vi "Eurotherm_2023_Module.vi"(3 "SP":bool=TRUE, 4 "Decimales":u16(ring)=1 items=["0"=1, "1"=10, "2"=100], 5 "Eurotherm (T:Enable)":bool=TRUE, 7 "Command":T3, 8 "error in (no error)":errorcluster, 9 "Value":dbl format="%04.1g", 10 "Address":T1(ring), 11 "VISA resource name":refnum<visa-resource-name>) -> (0 "error out":errorcluster, 2 "Eurotherm":T2)   [LabVIEW 2017]
uses:
  Eurotherm_2023_Module.ctl
  <vilib>/Instr/_visa.llb/VISA Configure Serial Port (Instr).vi
panel:
  out "String Read":string
  out "String Write":string
  # "NUEVO MODULO VI\nQUE INCORPORA LÍMITES DE SALIDA"
  # "Eurotherm New Module"
  # "Input Data"
  # "Local Data"
  # "Output Data"
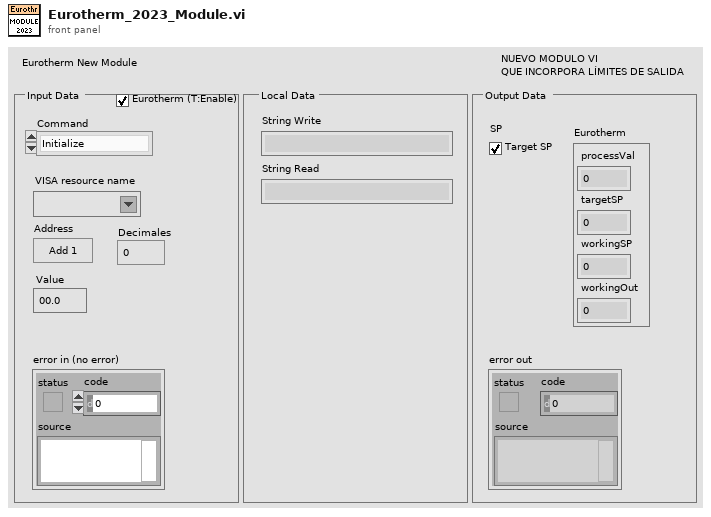
[diagram p1: front panel]
types:
  T1 = enum16{"Add 1", "Add 2", "Add 3", "Add 10", "Add 11", "Add 12", "Add 13"}
  T2 = cluster{"processVal":dbl, "targetSP":dbl, "workingSP":dbl, "workingOut":dbl}
  T3 = typedef "Eurotherm_2023_Module.ctl" = enum16{"Initialize", "Write setpoint", "Read data", "Write ramp rate", "Set constante proporcional", "Set constante integral", "Set constante diferencial", "Set ouput limit LOW", "Set ouput limit HIGH", "Shutdown"}
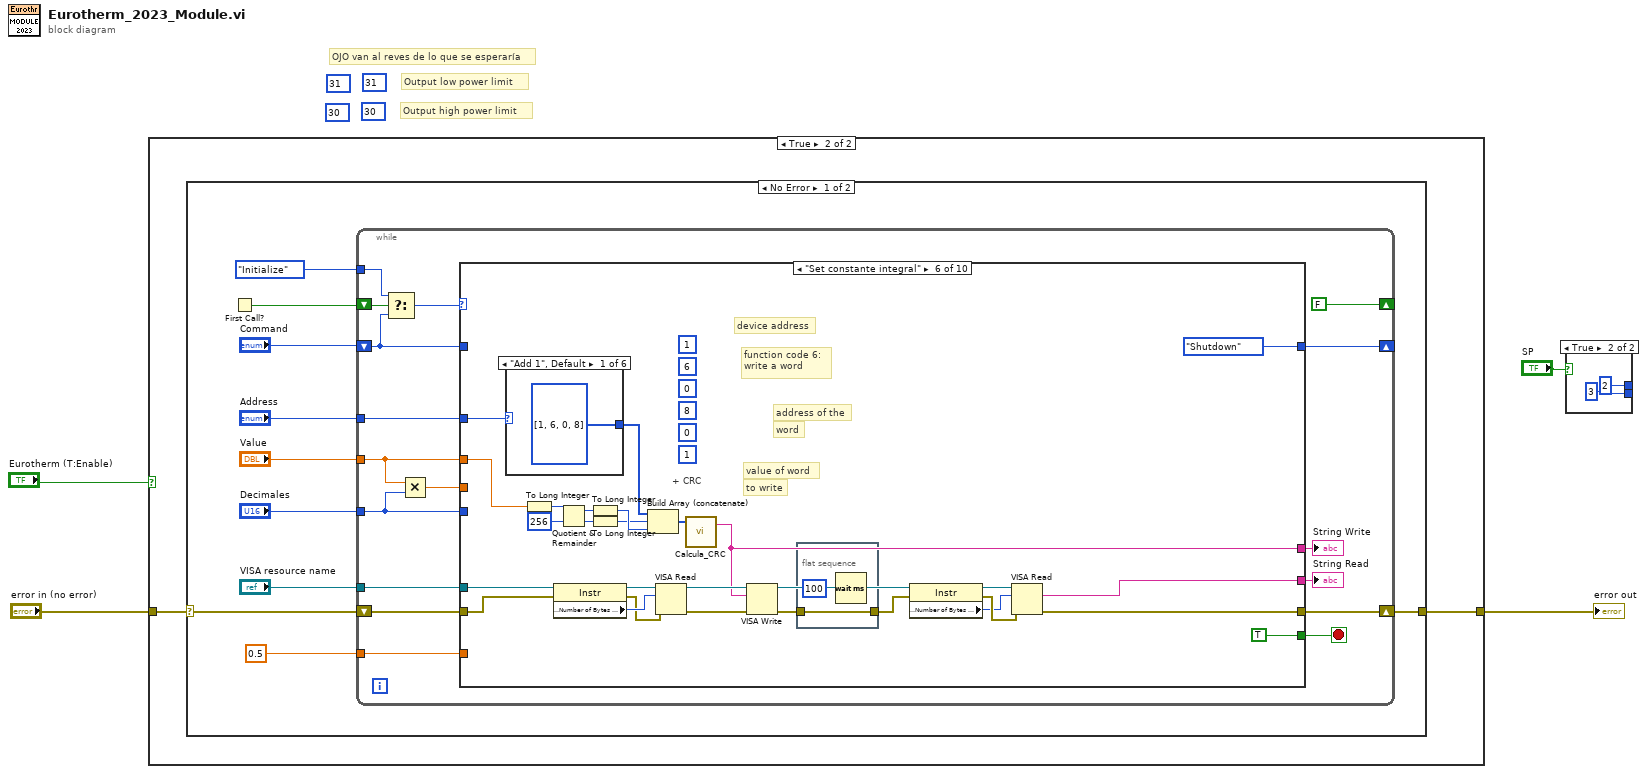
[diagram p0: block diagram]
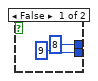
[diagram p2: hidden frame]
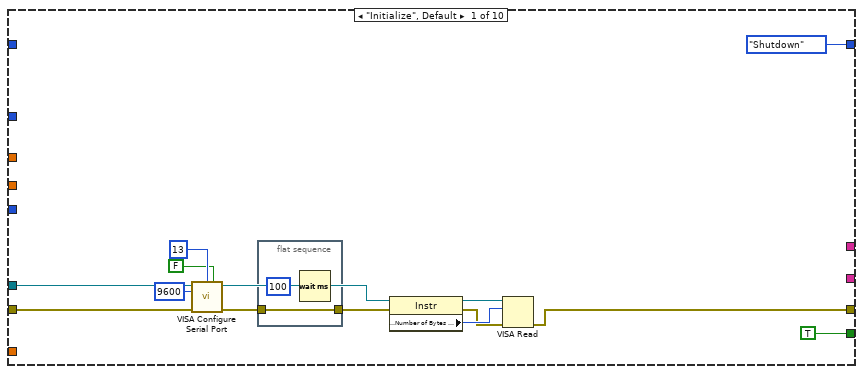
[diagram p4: hidden frame]
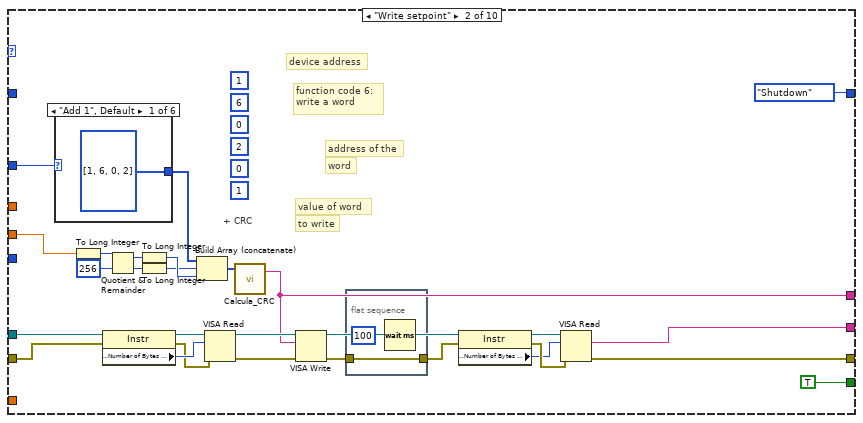
[diagram p5: hidden frame]
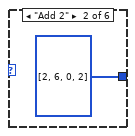
[diagram p6: hidden frame]
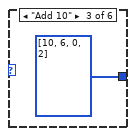
[diagram p7: hidden frame]
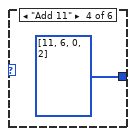
[diagram p8: hidden frame]
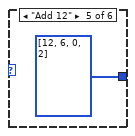
[diagram p9: hidden frame]
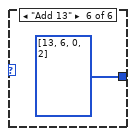
[diagram p10: hidden frame]
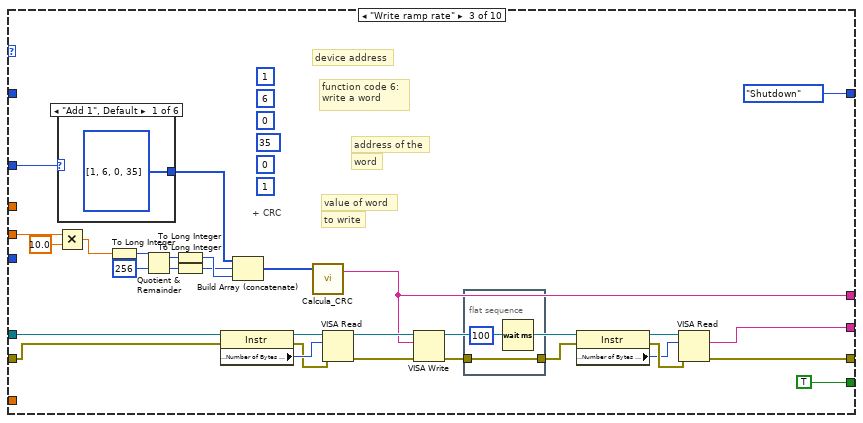
[diagram p11: hidden frame]
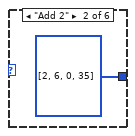
[diagram p12: hidden frame]
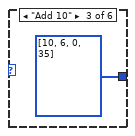
[diagram p13: hidden frame]
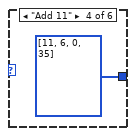
[diagram p14: hidden frame]
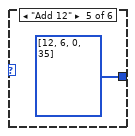
[diagram p15: hidden frame]
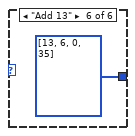
[diagram p16: hidden frame]
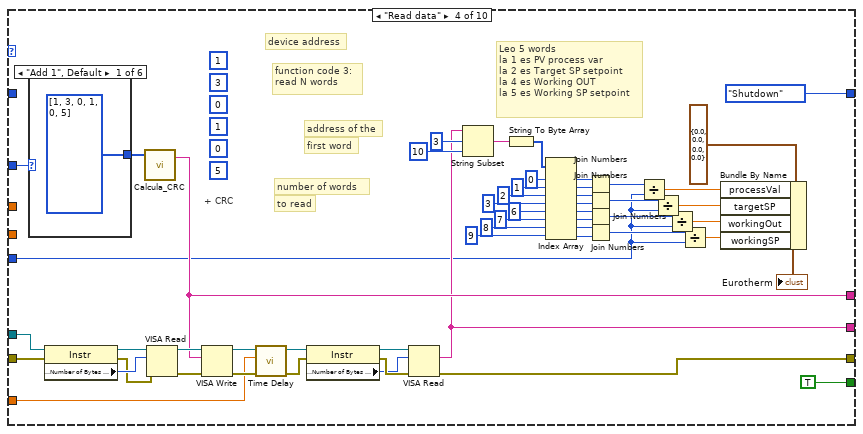
[diagram p17: hidden frame]
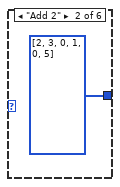
[diagram p18: hidden frame]
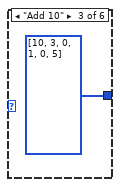
[diagram p19: hidden frame]
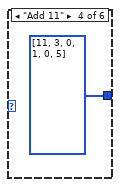
[diagram p20: hidden frame]
diagram:
  (unwired) u8 30
  (unwired) u8 31
  (unwired) u8 30
  (unwired) u8 31
  # "OJO van al reves de lo que se esperaría"
  # "Output high power limit"
  # "Output low power limit"
  n1 = case shown="True" "Eurotherm (T:Enable)" {
    tunnel: "error in (no error)" -> [w5 w7]
    tunnel: [w5 w6] -> w3
    frame False {
    }
    frame True {
      n2 = case shown="No Error" w7 {
        selector: w7 -> [w16 w368]
        tunnel: [w15 w368] -> w6
        frame No Error {
          n3 = First Call?() -> (First Call?: T/F=w17:bool)
          n4 = while {
            shift-right: [w29] -> _
            shift-left: "Command" -> [w30]
            shift-right: [w27] -> w15
            shift-left: w16 -> [w26]
            shift-right: [FALSE ("First Call?: T/F")] -> _
            shift-left: w17 -> [w34]
            tunnel: Eurotherm_2023_Module."Initialize" ("Command") -> [w33]
            tunnel: "Address" -> [w23]
            tunnel: "Value" -> [w20]
            tunnel: "Decimales" -> [w22]
            tunnel: "VISA resource name" -> [w19]
            tunnel: 0.5 ("milliseconds to wait") -> [w18]
            stop <- w28 stop-if-true
            n5 = Select(t=w33, s=w34, f=w30) -> (s? t:f=w31:T3)
            n6 = Multiply(x=w20, y=w22) -> (x*y=w21:dbl)
            n7 = case shown="\"Set constante integral\"" w31 {
              tunnel: w30 -> [_ _ _ _ _ _ _ _ _ _]
              tunnel: [Eurotherm_2023_Module."Shutdown" ("Command") Eurotherm_2023_Module."Shutdown" ("Command") Eurotherm_2023_Module."Shutdown" ("Command") Eurotherm_2023_Module."Shutdown" ("Command") Eurotherm_2023_Module."Shutdown" ("Command") Eurotherm_2023_Module."Shutdown" ("Command") Eurotherm_2023_Module."Shutdown" ("Command") Eurotherm_2023_Module."Shutdown" ("Command") Eurotherm_2023_Module."Shutdown" ("Command") Eurotherm_2023_Module."Shutdown" ("Command")] -> w29
              tunnel: [TRUE ("First Call?: T/F") TRUE ("First Call?: T/F") TRUE ("First Call?: T/F") TRUE ("First Call?: T/F") TRUE ("First Call?: T/F") TRUE ("First Call?: T/F") TRUE ("First Call?: T/F") TRUE ("First Call?: T/F") TRUE ("First Call?: T/F") TRUE ("First Call?: T/F")] -> w28
              tunnel: [w38 w58 w93 w154 w190 w226 w262 w298 w334 w364] -> w27
              tunnel: w26 -> [w39 w59 w96 w165 w191 w227 w263 w299 w335 w365]
              tunnel: w19 -> [w36 w57 w97 w164 w189 w225 w261 w297 w333 w366]
              tunnel: [_ w56 w92 w155 w188 w224 w260 w296 w332 _] -> w25
              tunnel: [_ w55 w91 w163 w187 w223 w259 w295 w331 _] -> w24
              tunnel: w23 -> [_ w53 w95 w176 w185 w221 w257 w293 w329 _]
              tunnel: w21 -> [_ w52 w90 _ _ _ _ _ _ _]
              tunnel: w22 -> [_ _ _ w132 _ _ _ _ _ _]
              tunnel: w20 -> [_ _ _ _ w184 w220 w256 w292 w328 _]
              tunnel: w18 -> [_ _ _ w141 _ _ _ _ _ _]
              frame "Initialize", Default {
                n8 = call-poly "VISA Configure Serial Port"("VISA resource name"=w36, "termination char\n(0xA = '\\n' = LF)"=u8 13 ("termination char\n(0xA = '\\n' = LF)"), "Enable Termination\nChar (T)"=FALSE ("Enable Termination\nChar (T)"), "baud rate (9600)"=u32 9600, "error in (no error)"=w39) -> ("VISA resource name out"=w40:refnum<visa-resource-name>, "error out"=w41:errorcluster)  [unwired: 9 in]
                n9 = flat-sequence {
                  tunnel: w41 -> [w49]
                  tunnel: [w49] -> w48
                  frame #0 {
                    n10 = Wait (ms)(milliseconds to wait=u32 100) -> ()  [unwired: 1 out]
                  }
                }
                n11 = property class="Instr"(reference=w40, error in=w48) -> (reference out=w45:refnum<visa-resource-name>, error out=w46:errorcluster, "Serial Settings:Number of Bytes at Serial Port"=w47:u32)
                n12 = VISA Read(VISA resource name=w45, byte count=w47, error in (no error)=w46) -> (error out=w38:errorcluster)  [unwired: 3 out]
              }
              frame "Write setpoint" {
                (unwired) 1
                (unwired) u8 0
                (unwired) 2
                (unwired) u8 0
                (unwired) 6
                (unwired) u8 1
                # "+ CRC"
                # "to write"
                # "value of word"
                # "word"
                # "address of the"
                # "function code 6:\nwrite a word"
                # "device address"
                n13 = case shown="\"Add 1\", Default" w53 {
                  tunnel: [u8[] [1, 6, 0, 2] ("Message Data") u8[] [2, 6, 0, 2] ("Message Data") u8[] [10, 6, 0, 2] ("Message Data") u8[] [11, 6, 0, 2] ("Message Data") u8[] [12, 6, 0, 2] ("Message Data") u8[] [13, 6, 0, 2] ("Message Data")] -> w78
                  frame "Add 1", Default {
                  }
                  frame "Add 2" {
                  }
                  frame "Add 10" {
                  }
                  frame "Add 11" {
                  }
                  frame "Add 12" {
                  }
                  frame "Add 13" {
                  }
                }
                n14 = To Long Integer(number=w52) -> (32bit integer=w77:i32)
                n15 = property class="Instr"(reference=w57, error in=w59) -> (reference out=w60:refnum<visa-resource-name>, error out=w61:errorcluster, "Serial Settings:Number of Bytes at Serial Port"=w62:u32)
                n16 = Quotient & Remainder(x=w77, y=256) -> (x-y*floor(x/y)=w72:i32, floor(x/y)=w73:i32)
                n17 = To Long Integer(number=w72) -> (32bit integer=w75:i32)
                n18 = To Long Integer(number=w73) -> (32bit integer=w74:i32)
                n19 = Build Array (concatenate)(w78, w74, w75) -> (w76:i32[])
                n20 = VISA Read(VISA resource name=w60, byte count=w62, error in (no error)=w61) -> (VISA resource name out=w69:refnum<visa-resource-name>, error out=w68:errorcluster)  [unwired: 2 out]
                n21 = call "Calcula_CRC.vi"("Message Data"=w76) -> ("String"=w55:string)  [unwired: 2 in, 1 out]
                n22 = VISA Write(VISA resource name=w69, write buffer=w55, error in (no error)=w68) -> (VISA resource name out=w70:refnum<visa-resource-name>, error out=w67:errorcluster)  [unwired: 1 out]
                n23 = flat-sequence {
                  tunnel: w67 -> [w79]
                  tunnel: [w79] -> w66
                  frame #0 {
                    n24 = Wait (ms)(milliseconds to wait=u32 100) -> ()  [unwired: 1 out]
                  }
                }
                n25 = property class="Instr"(reference=w70, error in=w66) -> (reference out=w65:refnum<visa-resource-name>, error out=w64:errorcluster, "Serial Settings:Number of Bytes at Serial Port"=w63:u32)
                n26 = VISA Read(VISA resource name=w65, byte count=w63, error in (no error)=w64) -> (read buffer=w56:string, error out=w58:errorcluster)  [unwired: 2 out]
              }
              frame "Write ramp rate" {
                (unwired) 1
                (unwired) u8 0
                (unwired) 35
                (unwired) u8 0
                (unwired) 6
                (unwired) u8 1
                # "+ CRC"
                # "to write"
                # "value of word"
                # "word"
                # "address of the"
                # "function code 6:\nwrite a word"
                # "device address"
                n27 = Multiply(x=w90, y=10.0) -> (x*y=w89:dbl)
                n28 = case shown="\"Add 1\", Default" w95 {
                  tunnel: [u8[] [1, 6, 0, 35] ("Message Data") u8[] [2, 6, 0, 35] ("Message Data") u8[] [10, 6, 0, 35] ("Message Data") u8[] [11, 6, 0, 35] ("Message Data") u8[] [12, 6, 0, 35] ("Message Data") u8[] [13, 6, 0, 35] ("Message Data")] -> w116
                  frame "Add 1", Default {
                  }
                  frame "Add 2" {
                  }
                  frame "Add 10" {
                  }
                  frame "Add 11" {
                  }
                  frame "Add 12" {
                  }
                  frame "Add 13" {
                  }
                }
                n29 = To Long Integer(number=w89) -> (32bit integer=w115:i32)
                n30 = Quotient & Remainder(x=w115, y=256) -> (x-y*floor(x/y)=w110:i32, floor(x/y)=w111:i32)
                n31 = To Long Integer(number=w110) -> (32bit integer=w113:i32)
                n32 = To Long Integer(number=w111) -> (32bit integer=w112:i32)
                n33 = property class="Instr"(reference=w97, error in=w96) -> (reference out=w98:refnum<visa-resource-name>, error out=w99:errorcluster, "Serial Settings:Number of Bytes at Serial Port"=w100:u32)
                n34 = Build Array (concatenate)(w116, w112, w113) -> (w114:i32[])
                n35 = call "Calcula_CRC.vi"("Message Data"=w114) -> ("String"=w91:string)  [unwired: 2 in, 1 out]
                n36 = VISA Read(VISA resource name=w98, byte count=w100, error in (no error)=w99) -> (VISA resource name out=w107:refnum<visa-resource-name>, error out=w106:errorcluster)  [unwired: 2 out]
                n37 = VISA Write(VISA resource name=w107, write buffer=w91, error in (no error)=w106) -> (VISA resource name out=w108:refnum<visa-resource-name>, error out=w105:errorcluster)  [unwired: 1 out]
                n38 = flat-sequence {
                  tunnel: w105 -> [w117]
                  tunnel: [w117] -> w104
                  frame #0 {
                    n39 = Wait (ms)(milliseconds to wait=u32 100) -> ()  [unwired: 1 out]
                  }
                }
                n40 = property class="Instr"(reference=w108, error in=w104) -> (reference out=w103:refnum<visa-resource-name>, error out=w102:errorcluster, "Serial Settings:Number of Bytes at Serial Port"=w101:u32)
                n41 = VISA Read(VISA resource name=w103, byte count=w101, error in (no error)=w102) -> (read buffer=w92:string, error out=w93:errorcluster)  [unwired: 2 out]
              }
              frame "Read data" {
                (unwired) u8 5
                (unwired) u8 0
                (unwired) u8 1
                (unwired) u8 0
                (unwired) u8 3
                (unwired) u8 1
                # "+ CRC"
                # "to read"
                # "number of words"
                # "first word"
                # "address of the"
                # "function code 3:\nread N words"
                # "device address"
                # "Leo 5 words\nla 1 es PV process var\nla 2 es Target SP setpoint\nla 4 es Working OUT\nla 5 es Working SP setpoint"
                n42 = case shown="\"Add 1\", Default" w176 {
                  tunnel: [u8[] [1, 3, 0, 1, 0, 5] ("Message Data") u8[] [2, 3, 0, 1, 0, 5] ("Message Data") u8[] [10, 3, 0, 1, 0, 5] ("Message Data") u8[] [11, 3, 0, 1, 0, 5] ("Message Data") u8[] [12, 3, 0, 1, 0, 5] ("Message Data") u8[] [13, 3, 0, 1, 0, 5] ("Message Data")] -> w175
                  frame "Add 1", Default {
                  }
                  frame "Add 2" {
                  }
                  frame "Add 10" {
                  }
                  frame "Add 11" {
                  }
                  frame "Add 12" {
                  }
                  frame "Add 13" {
                  }
                }
                n43 = property class="Instr"(reference=w164, error in=w165) -> (reference out=w166:refnum<visa-resource-name>, error out=w167:errorcluster, "Serial Settings:Number of Bytes at Serial Port"=w168:u32)
                n44 = call "Calcula_CRC.vi"("Message Data"=w175) -> ("String"=w163:string)  [unwired: 2 in, 1 out]
                n45 = VISA Read(VISA resource name=w166, byte count=w168, error in (no error)=w167) -> (VISA resource name out=w173:refnum<visa-resource-name>, error out=w172:errorcluster)  [unwired: 2 out]
                n46 = VISA Write(VISA resource name=w173, write buffer=w163, error in (no error)=w172) -> (VISA resource name out=w174:refnum<visa-resource-name>, error out=w143:errorcluster)  [unwired: 1 out]
                n47 = call "Time Delay"("error in (no error)"=w143, "Delay Time (s)"=w141) -> ("error out"=w142:errorcluster)  [unwired: 9 in]
                n48 = property class="Instr"(reference=w174, error in=w142) -> (reference out=w171:refnum<visa-resource-name>, error out=w170:errorcluster, "Serial Settings:Number of Bytes at Serial Port"=w169:u32)
                n49 = VISA Read(VISA resource name=w171, byte count=w169, error in (no error)=w170) -> (read buffer=w155:string, error out=w154:errorcluster)  [unwired: 2 out]
                n50 = String Subset(string=w155, offset (0)=3, length (rest)=10 ("length (rest)")) -> (substring=w156:string)
                n51 = String To Byte Array(string=w156) -> (unsigned byte array=w159:u8[])
                n52 = Index Array(array=w159, index #1=0 ("index"), index #2=1 ("index"), index #3=2 ("index"), index #4=3 ("index"), index #5=6 ("index"), index #6=7 ("index"), index #7=8 ("index"), index #8=9 ("index")) -> (element #1=w147:u8, element #2=w146:u8, element #3=w145:u8, element #4=w144:u8, element #5=w140:u8, element #6=w139:u8, element #7=w138:u8, element #8=w137:u8)
                n53 = Join Numbers(hi=w147, lo=w146) -> ((hi.lo)=w136:u16)
                n54 = Join Numbers(hi=w145, lo=w144) -> ((hi.lo)=w135:u16)
                n55 = Join Numbers(hi=w140, lo=w139) -> ((hi.lo)=w134:u16)
                n56 = Join Numbers(hi=w138, lo=w137) -> ((hi.lo)=w133:u16)
                n57 = Divide(x=w136, y=w132) -> (x/y=w126:dbl)
                n58 = Divide(x=w135, y=w132) -> (x/y=w127:dbl)
                n59 = Divide(x=w134, y=w132) -> (x/y=w128:dbl)
                n60 = Divide(x=w133, y=w132) -> (x/y=w129:dbl)
                n61 = Bundle By Name(cluster=T2 {"processVal"=0.0, "targetSP"=0.0, "workingSP"=0.0, "workingOut"=0.0} ("Eurotherm"), "processVal"=w126, "targetSP"=w127, "workingOut"=w128, "workingSP"=w129) -> (→"Eurotherm":T2)
              }
              frame "Set constante proporcional" {
                (unwired) 1
                (unwired) u8 0
                (unwired) 6
                (unwired) u8 0
                (unwired) 6
                (unwired) u8 1
                # "+ CRC"
                # "to write"
                # "value of word"
                # "word"
                # "address of the"
                # "function code 6:\nwrite a word"
                # "device address"
                n62 = case shown="\"Add 1\", Default" w185 {
                  tunnel: [u8[] [1, 6, 0, 6] ("Message Data") u8[] [2, 6, 0, 6] ("Message Data") u8[] [10, 6, 0, 6] ("Message Data") u8[] [11, 6, 0, 6] ("Message Data") u8[] [12, 6, 0, 6] ("Message Data") u8[] [13, 6, 0, 6] ("Message Data")] -> w210
                  frame "Add 1", Default {
                  }
                  frame "Add 2" {
                  }
                  frame "Add 10" {
                  }
                  frame "Add 11" {
                  }
                  frame "Add 12" {
                  }
                  frame "Add 13" {
                  }
                }
                n63 = To Long Integer(number=w184) -> (32bit integer=w209:i32)
                n64 = property class="Instr"(reference=w189, error in=w191) -> (reference out=w192:refnum<visa-resource-name>, error out=w193:errorcluster, "Serial Settings:Number of Bytes at Serial Port"=w194:u32)
                n65 = Quotient & Remainder(x=w209, y=256) -> (x-y*floor(x/y)=w204:i32, floor(x/y)=w205:i32)
                n66 = To Long Integer(number=w204) -> (32bit integer=w207:i32)
                n67 = To Long Integer(number=w205) -> (32bit integer=w206:i32)
                n68 = Build Array (concatenate)(w210, w206, w207) -> (w208:i32[])
                n69 = VISA Read(VISA resource name=w192, byte count=w194, error in (no error)=w193) -> (VISA resource name out=w201:refnum<visa-resource-name>, error out=w200:errorcluster)  [unwired: 2 out]
                n70 = call "Calcula_CRC.vi"("Message Data"=w208) -> ("String"=w187:string)  [unwired: 2 in, 1 out]
                n71 = VISA Write(VISA resource name=w201, write buffer=w187, error in (no error)=w200) -> (VISA resource name out=w202:refnum<visa-resource-name>, error out=w199:errorcluster)  [unwired: 1 out]
                n72 = flat-sequence {
                  tunnel: w199 -> [w211]
                  tunnel: [w211] -> w198
                  frame #0 {
                    n73 = Wait (ms)(milliseconds to wait=u32 100) -> ()  [unwired: 1 out]
                  }
                }
                n74 = property class="Instr"(reference=w202, error in=w198) -> (reference out=w197:refnum<visa-resource-name>, error out=w196:errorcluster, "Serial Settings:Number of Bytes at Serial Port"=w195:u32)
                n75 = VISA Read(VISA resource name=w197, byte count=w195, error in (no error)=w196) -> (read buffer=w188:string, error out=w190:errorcluster)  [unwired: 2 out]
              }
              frame "Set constante integral" {
                (unwired) 1
                (unwired) u8 0
                (unwired) 8
                (unwired) u8 0
                (unwired) 6
                (unwired) u8 1
                # "+ CRC"
                # "to write"
                # "value of word"
                # "word"
                # "address of the"
                # "function code 6:\nwrite a word"
                # "device address"
                n76 = case shown="\"Add 1\", Default" w221 {
                  tunnel: [u8[] [1, 6, 0, 8] ("Message Data") u8[] [2, 6, 0, 8] ("Message Data") u8[] [10, 6, 0, 8] ("Message Data") u8[] [11, 6, 0, 8] ("Message Data") u8[] [12, 6, 0, 8] ("Message Data") u8[] [13, 6, 0, 8] ("Message Data")] -> w246
                  frame "Add 1", Default {
                  }
                  frame "Add 2" {
                  }
                  frame "Add 10" {
                  }
                  frame "Add 11" {
                  }
                  frame "Add 12" {
                  }
                  frame "Add 13" {
                  }
                }
                n77 = To Long Integer(number=w220) -> (32bit integer=w245:i32)
                n78 = property class="Instr"(reference=w225, error in=w227) -> (reference out=w228:refnum<visa-resource-name>, error out=w229:errorcluster, "Serial Settings:Number of Bytes at Serial Port"=w230:u32)
                n79 = Quotient & Remainder(x=w245, y=256) -> (x-y*floor(x/y)=w240:i32, floor(x/y)=w241:i32)
                n80 = To Long Integer(number=w240) -> (32bit integer=w243:i32)
                n81 = To Long Integer(number=w241) -> (32bit integer=w242:i32)
                n82 = Build Array (concatenate)(w246, w242, w243) -> (w244:i32[])
                n83 = VISA Read(VISA resource name=w228, byte count=w230, error in (no error)=w229) -> (VISA resource name out=w237:refnum<visa-resource-name>, error out=w236:errorcluster)  [unwired: 2 out]
                n84 = call "Calcula_CRC.vi"("Message Data"=w244) -> ("String"=w223:string)  [unwired: 2 in, 1 out]
                n85 = VISA Write(VISA resource name=w237, write buffer=w223, error in (no error)=w236) -> (VISA resource name out=w238:refnum<visa-resource-name>, error out=w235:errorcluster)  [unwired: 1 out]
                n86 = flat-sequence {
                  tunnel: w235 -> [w247]
                  tunnel: [w247] -> w234
                  frame #0 {
                    n87 = Wait (ms)(milliseconds to wait=u32 100) -> ()  [unwired: 1 out]
                  }
                }
                n88 = property class="Instr"(reference=w238, error in=w234) -> (reference out=w233:refnum<visa-resource-name>, error out=w232:errorcluster, "Serial Settings:Number of Bytes at Serial Port"=w231:u32)
                n89 = VISA Read(VISA resource name=w233, byte count=w231, error in (no error)=w232) -> (read buffer=w224:string, error out=w226:errorcluster)  [unwired: 2 out]
              }
              frame "Set constante diferencial" {
                (unwired) 1
                (unwired) u8 0
                (unwired) 9
                (unwired) u8 0
                (unwired) 6
                (unwired) u8 1
                # "+ CRC"
                # "to write"
                # "value of word"
                # "word"
                # "address of the"
                # "function code 6:\nwrite a word"
                # "device address"
                n90 = case shown="\"Add 1\", Default" w257 {
                  tunnel: [u8[] [1, 6, 0, 9] ("Message Data") u8[] [2, 6, 0, 9] ("Message Data") u8[] [10, 6, 0, 9] ("Message Data") u8[] [11, 6, 0, 9] ("Message Data") u8[] [12, 6, 0, 9] ("Message Data") u8[] [13, 6, 0, 9] ("Message Data")] -> w282
                  frame "Add 1", Default {
                  }
                  frame "Add 2" {
                  }
                  frame "Add 10" {
                  }
                  frame "Add 11" {
                  }
                  frame "Add 12" {
                  }
                  frame "Add 13" {
                  }
                }
                n91 = To Long Integer(number=w256) -> (32bit integer=w281:i32)
                n92 = property class="Instr"(reference=w261, error in=w263) -> (reference out=w264:refnum<visa-resource-name>, error out=w265:errorcluster, "Serial Settings:Number of Bytes at Serial Port"=w266:u32)
                n93 = Quotient & Remainder(x=w281, y=256) -> (x-y*floor(x/y)=w276:i32, floor(x/y)=w277:i32)
                n94 = To Long Integer(number=w276) -> (32bit integer=w279:i32)
                n95 = To Long Integer(number=w277) -> (32bit integer=w278:i32)
                n96 = Build Array (concatenate)(w282, w278, w279) -> (w280:i32[])
                n97 = VISA Read(VISA resource name=w264, byte count=w266, error in (no error)=w265) -> (VISA resource name out=w273:refnum<visa-resource-name>, error out=w272:errorcluster)  [unwired: 2 out]
                n98 = call "Calcula_CRC.vi"("Message Data"=w280) -> ("String"=w259:string)  [unwired: 2 in, 1 out]
                n99 = VISA Write(VISA resource name=w273, write buffer=w259, error in (no error)=w272) -> (VISA resource name out=w274:refnum<visa-resource-name>, error out=w271:errorcluster)  [unwired: 1 out]
                n100 = flat-sequence {
                  tunnel: w271 -> [w283]
                  tunnel: [w283] -> w270
                  frame #0 {
                    n101 = Wait (ms)(milliseconds to wait=u32 100) -> ()  [unwired: 1 out]
                  }
                }
                n102 = property class="Instr"(reference=w274, error in=w270) -> (reference out=w269:refnum<visa-resource-name>, error out=w268:errorcluster, "Serial Settings:Number of Bytes at Serial Port"=w267:u32)
                n103 = VISA Read(VISA resource name=w269, byte count=w267, error in (no error)=w268) -> (read buffer=w260:string, error out=w262:errorcluster)  [unwired: 2 out]
              }
              frame "Set ouput limit LOW" {
                (unwired) 1
                (unwired) u8 0
                (unwired) 31
                (unwired) u8 0
                (unwired) 6
                (unwired) u8 1
                # "+ CRC"
                # "to write"
                # "value of word"
                # "word"
                # "address of the"
                # "function code 6:\nwrite a word"
                # "device address"
                n104 = case shown="\"Add 1\", Default" w293 {
                  tunnel: [u8[] [1, 6, 0, 31] ("Message Data") u8[] [2, 6, 0, 31] ("Message Data") u8[] [10, 6, 0, 31] ("Message Data") u8[] [11, 6, 0, 31] ("Message Data") u8[] [12, 6, 0, 31] ("Message Data") u8[] [13, 6, 0, 31] ("Message Data")] -> w318
                  frame "Add 1", Default {
                  }
                  frame "Add 2" {
                  }
                  frame "Add 10" {
                  }
                  frame "Add 11" {
                  }
                  frame "Add 12" {
                  }
                  frame "Add 13" {
                  }
                }
                n105 = To Long Integer(number=w292) -> (32bit integer=w317:i32)
                n106 = property class="Instr"(reference=w297, error in=w299) -> (reference out=w300:refnum<visa-resource-name>, error out=w301:errorcluster, "Serial Settings:Number of Bytes at Serial Port"=w302:u32)
                n107 = Quotient & Remainder(x=w317, y=256) -> (x-y*floor(x/y)=w312:i32, floor(x/y)=w313:i32)
                n108 = To Long Integer(number=w312) -> (32bit integer=w315:i32)
                n109 = To Long Integer(number=w313) -> (32bit integer=w314:i32)
                n110 = Build Array (concatenate)(w318, w314, w315) -> (w316:i32[])
                n111 = VISA Read(VISA resource name=w300, byte count=w302, error in (no error)=w301) -> (VISA resource name out=w309:refnum<visa-resource-name>, error out=w308:errorcluster)  [unwired: 2 out]
                n112 = call "Calcula_CRC.vi"("Message Data"=w316) -> ("String"=w295:string)  [unwired: 2 in, 1 out]
                n113 = VISA Write(VISA resource name=w309, write buffer=w295, error in (no error)=w308) -> (VISA resource name out=w310:refnum<visa-resource-name>, error out=w307:errorcluster)  [unwired: 1 out]
                n114 = flat-sequence {
                  tunnel: w307 -> [w319]
                  tunnel: [w319] -> w306
                  frame #0 {
                    n115 = Wait (ms)(milliseconds to wait=u32 100) -> ()  [unwired: 1 out]
                  }
                }
                n116 = property class="Instr"(reference=w310, error in=w306) -> (reference out=w305:refnum<visa-resource-name>, error out=w304:errorcluster, "Serial Settings:Number of Bytes at Serial Port"=w303:u32)
                n117 = VISA Read(VISA resource name=w305, byte count=w303, error in (no error)=w304) -> (read buffer=w296:string, error out=w298:errorcluster)  [unwired: 2 out]
              }
              frame "Set ouput limit HIGH" {
                (unwired) 1
                (unwired) u8 0
                (unwired) 30
                (unwired) u8 0
                (unwired) 6
                (unwired) u8 1
                # "+ CRC"
                # "to write"
                # "value of word"
                # "word"
                # "address of the"
                # "function code 6:\nwrite a word"
                # "device address"
                n118 = case shown="\"Add 1\", Default" w329 {
                  tunnel: [u8[] [1, 6, 0, 30] ("Message Data") u8[] [2, 6, 0, 30] ("Message Data") u8[] [10, 6, 0, 30] ("Message Data") u8[] [11, 6, 0, 30] ("Message Data") u8[] [12, 6, 0, 30] ("Message Data") u8[] [13, 6, 0, 30] ("Message Data")] -> w354
                  frame "Add 1", Default {
                  }
                  frame "Add 2" {
                  }
                  frame "Add 10" {
                  }
                  frame "Add 11" {
                  }
                  frame "Add 12" {
                  }
                  frame "Add 13" {
                  }
                }
                n119 = To Long Integer(number=w328) -> (32bit integer=w353:i32)
                n120 = property class="Instr"(reference=w333, error in=w335) -> (reference out=w336:refnum<visa-resource-name>, error out=w337:errorcluster, "Serial Settings:Number of Bytes at Serial Port"=w338:u32)
                n121 = Quotient & Remainder(x=w353, y=256) -> (x-y*floor(x/y)=w348:i32, floor(x/y)=w349:i32)
                n122 = To Long Integer(number=w348) -> (32bit integer=w351:i32)
                n123 = To Long Integer(number=w349) -> (32bit integer=w350:i32)
                n124 = Build Array (concatenate)(w354, w350, w351) -> (w352:i32[])
                n125 = VISA Read(VISA resource name=w336, byte count=w338, error in (no error)=w337) -> (VISA resource name out=w345:refnum<visa-resource-name>, error out=w344:errorcluster)  [unwired: 2 out]
                n126 = call "Calcula_CRC.vi"("Message Data"=w352) -> ("String"=w331:string)  [unwired: 2 in, 1 out]
                n127 = VISA Write(VISA resource name=w345, write buffer=w331, error in (no error)=w344) -> (VISA resource name out=w346:refnum<visa-resource-name>, error out=w343:errorcluster)  [unwired: 1 out]
                n128 = flat-sequence {
                  tunnel: w343 -> [w355]
                  tunnel: [w355] -> w342
                  frame #0 {
                    n129 = Wait (ms)(milliseconds to wait=u32 100) -> ()  [unwired: 1 out]
                  }
                }
                n130 = property class="Instr"(reference=w346, error in=w342) -> (reference out=w341:refnum<visa-resource-name>, error out=w340:errorcluster, "Serial Settings:Number of Bytes at Serial Port"=w339:u32)
                n131 = VISA Read(VISA resource name=w341, byte count=w339, error in (no error)=w340) -> (read buffer=w332:string, error out=w334:errorcluster)  [unwired: 2 out]
              }
              frame "Shutdown" {
                n132 = VISA Close(VISA resource name=w366, error in (no error)=w365) -> (error out=w364:errorcluster)
              }
            }
            "String Read" <- w25
            "String Write" <- w24
          }
        }
        frame Error {
        }
      }
    }
  }
  "error out" <- w3
  n133 = case shown="True" "SP" {
    tunnel: [8 ("index") 2 ("index")] -> _
    tunnel: [9 ("index") 3 ("index")] -> _
    frame False {
    }
    frame True {
    }
  }
